vi "RampVoltagewithDDSv6,FastPiezo.vi"(0 "Sample rate":dbl=500000.0, 2 "Ramp Samples":dbl, 3 "Ramp 1 Duration (ms)":dbl=500000.0, 4 "Plateau 1 (ms)":dbl, 5 "Ramp 2 Duration (ms)":dbl=500000.0, 7 "Delay 2 (ms)":dbl, 8 "Delay 1 (ms)":dbl, 9 "Ramp 3 Duration (ms)":dbl=500000.0, 11 "Plateau 2 (ms)":dbl, 13 "Ramp 4 Duration (ms)":dbl=500000.0, 16 "Ramp 4 Amplitude":dbl=500000.0, 17 "Ramp 2 Amplitude":dbl=500000.0, 18 "Ramp 3 Amplitude":dbl=500000.0, 19 "Ramp 1 Amplitude":dbl=500000.0) -> (14 "appended array":dbl[](array[numeric]))   [LabVIEW 2016]
panel:
  out "size(s) 2":i32
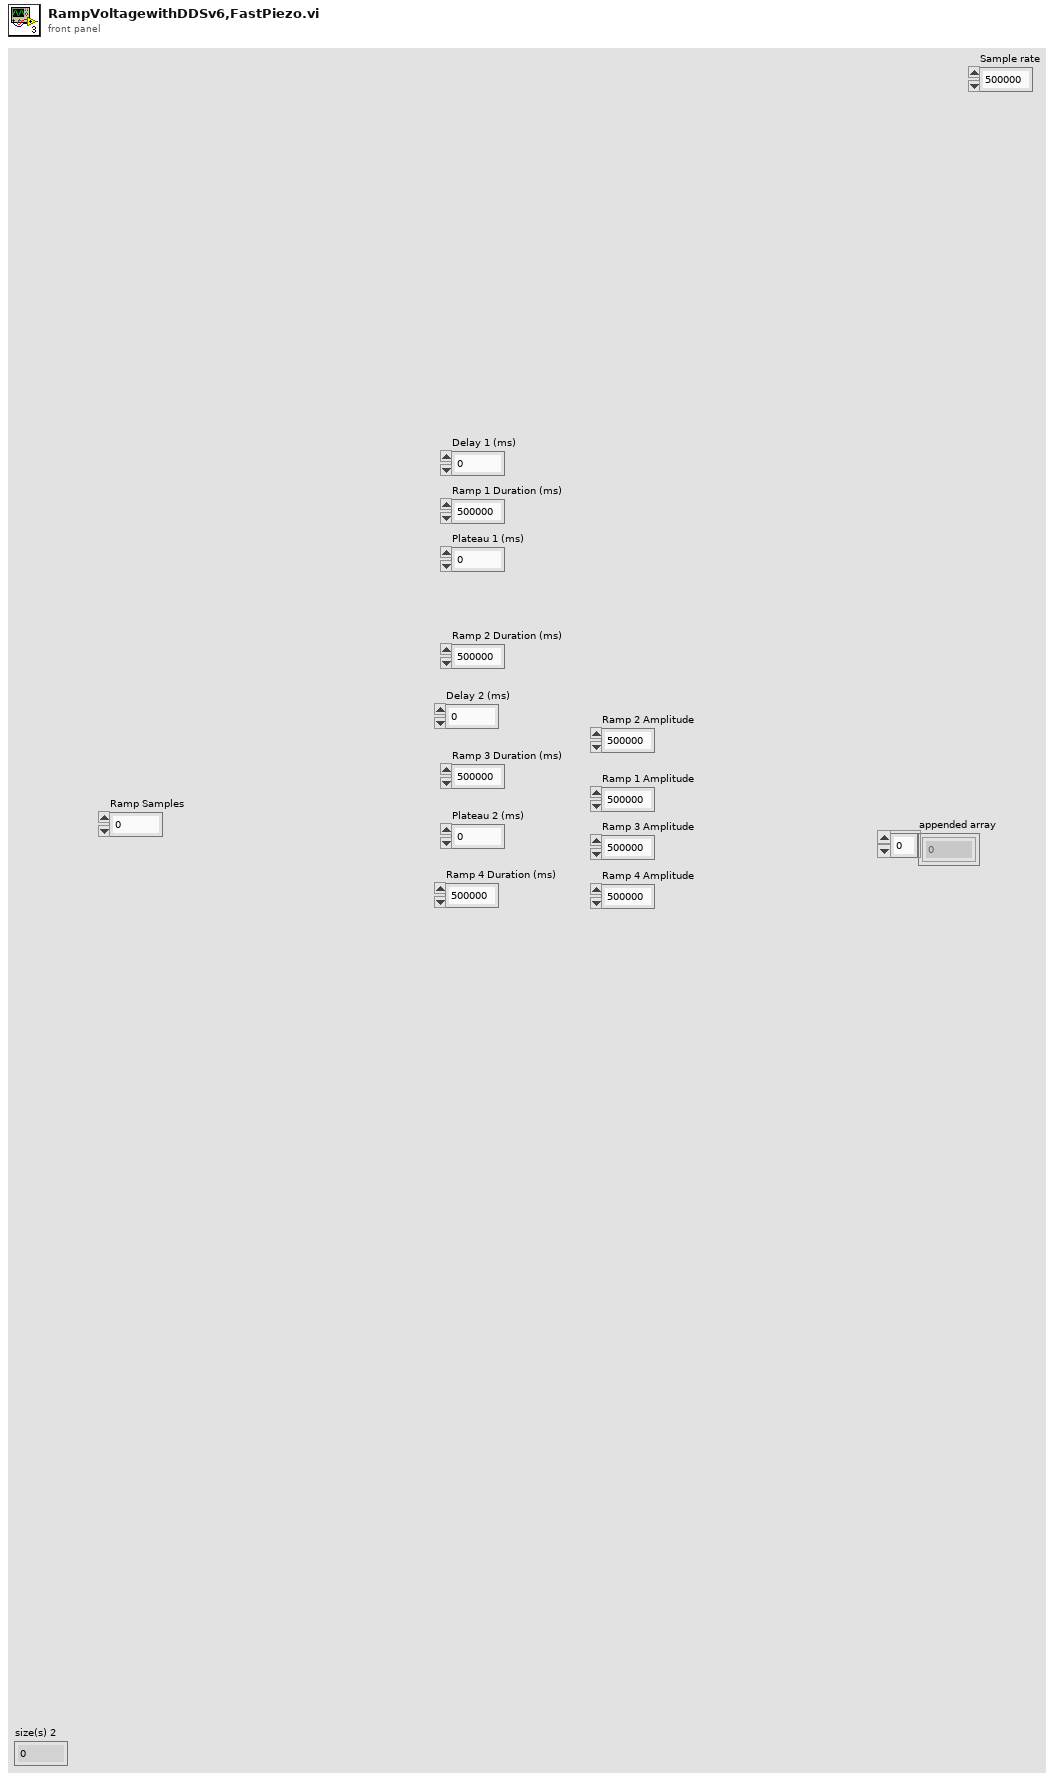
[diagram p1: front panel]
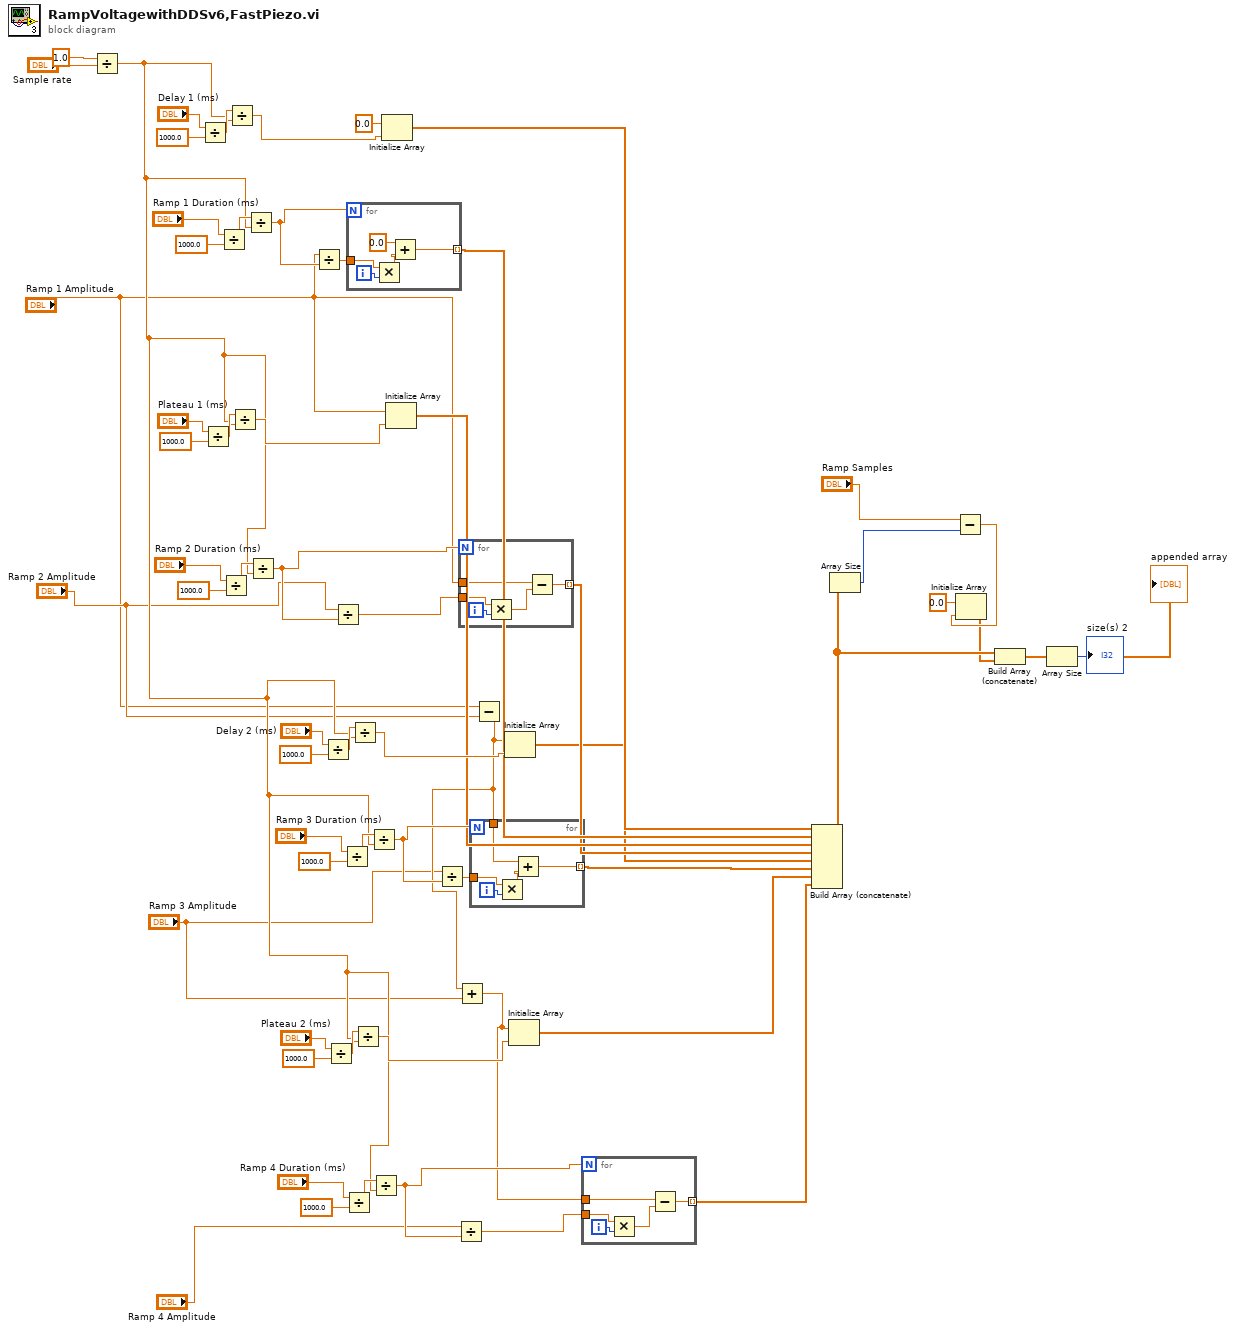
[diagram p0: block diagram]
diagram:
  n1 = Divide(x=1.0, y="Sample rate") -> (x/y=w23:dbl)
  n2 = Divide(x="Delay 1 (ms)", y=1000.0) -> (x/y=w58:dbl)
  n3 = Divide(x="Plateau 1 (ms)", y=1000.0) -> (x/y=w50:dbl)
  n4 = Divide(x="Ramp 1 Duration (ms)", y=1000.0) -> (x/y=w55:dbl)
  n5 = Divide(x="Ramp 2 Duration (ms)", y=1000.0) -> (x/y=w47:dbl)
  n6 = Divide(x=w58, y=w23) -> (x/y=w43:dbl)
  n7 = Divide(x=w50, y=w23) -> (x/y=w42:dbl)
  n8 = Divide(x=w55, y=w23) -> (x/y=w54:dbl)
  n9 = Divide(x=w47, y=w23) -> (x/y=w46:dbl)
  n10 = Divide(x="Ramp 1 Amplitude", y=w54) -> (x/y=w53:dbl)
  n11 = Divide(x="Delay 2 (ms)", y=1000.0) -> (x/y=w39:dbl)
  n12 = Divide(x="Plateau 2 (ms)", y=1000.0) -> (x/y=w31:dbl)
  n13 = Divide(x="Ramp 2 Amplitude", y=w46) -> (x/y=w45:dbl)
  n14 = Divide(x="Ramp 3 Duration (ms)", y=1000.0) -> (x/y=w36:dbl)
  n15 = Divide(x="Ramp 4 Duration (ms)", y=1000.0) -> (x/y=w28:dbl)
  n16 = for {
    N: w54 -> [_]
    tunnel: [w66] -> w21 mode=indexing
    tunnel: w53 -> [w64]
    i -> [w65]
    n17 = Multiply(x=w64, y=w65) -> (x*y=w63:dbl)
    n18 = Add(x=0.0 ("y"), y=w63) -> (x+y=w66:dbl)
  }
  n19 = Divide(x=w39, y=w23) -> (x/y=w25:dbl)
  n20 = Divide(x=w31, y=w23) -> (x/y=w24:dbl)
  n21 = Divide(x=w36, y=w23) -> (x/y=w35:dbl)
  n22 = Divide(x=w28, y=w23) -> (x/y=w27:dbl)
  n23 = Initialize Array(0.0 ("element"), w43) -> (w22:dbl[])
  n24 = Initialize Array("Ramp 1 Amplitude", w42) -> (w20:dbl[])
  n25 = Divide(x="Ramp 3 Amplitude", y=w35) -> (x/y=w34:dbl)
  n26 = Divide(x="Ramp 4 Amplitude", y=w27) -> (x/y=w26:dbl)
  n27 = for {
    N: w46 -> [_]
    tunnel: [w72] -> w19 mode=indexing
    tunnel: w45 -> [w70]
    tunnel: "Ramp 1 Amplitude" -> [w68]
    i -> [w71]
    n28 = Multiply(x=w70, y=w71) -> (x*y=w69:dbl)
    n29 = Subtract(x=w68, y=w69) -> (x-y=w72:dbl)
  }
  n30 = Subtract(x="Ramp 1 Amplitude", y="Ramp 2 Amplitude") -> (x-y=w4:dbl)
  n31 = Add(x=w4, y="Ramp 3 Amplitude") -> (x+y=w2:dbl)
  n32 = for {
    N: w35 -> [_]
    tunnel: [w77] -> w17 mode=indexing
    tunnel: w34 -> [w75]
    tunnel: w4 -> [w73]
    i -> [w76]
    n33 = Multiply(x=w75, y=w76) -> (x*y=w74:dbl)
    n34 = Add(x=w73, y=w74) -> (x+y=w77:dbl)
  }
  n35 = Initialize Array(w4, w25) -> (w18:dbl[])
  n36 = Initialize Array(w2, w24) -> (w16:dbl[])
  n37 = for {
    N: w27 -> [_]
    tunnel: [w82] -> w7 mode=indexing
    tunnel: w26 -> [w80]
    tunnel: w2 -> [w78]
    i -> [w81]
    n38 = Multiply(x=w80, y=w81) -> (x*y=w79:dbl)
    n39 = Subtract(x=w78, y=w79) -> (x-y=w82:dbl)
  }
  n40 = Build Array (concatenate)(w22, w21, w20, w19, w18, w17, w16, w7) -> (w11:dbl[])
  n41 = Array Size(array=w11) -> (size(s)=w14:i32)
  n42 = Subtract(x="Ramp Samples", y=w14) -> (x-y=w12:dbl)
  n43 = Initialize Array(0.0 ("element"), w12) -> (w10:dbl[])
  n44 = Build Array (concatenate)(w11, w10) -> (w8:dbl[])
  "appended array" <- w8
  n45 = Array Size(array=w8) -> (size(s)=→"size(s) 2":i32)
